vi "Parset_1.vi"(8 "error in (no error)":errorcluster, 11 "Programing Logic in":refnum<class "Programing Logic.lvclass">) -> (0 "error out":errorcluster, 3 "Programing Logic out":refnum<class "Programing Logic.lvclass">)   [LabVIEW 2014, in "Programing Logic.lvclass"]
uses:
  Programing Logic.lvclass
  Programing Logic.lvclass/Programing Logic.ctl
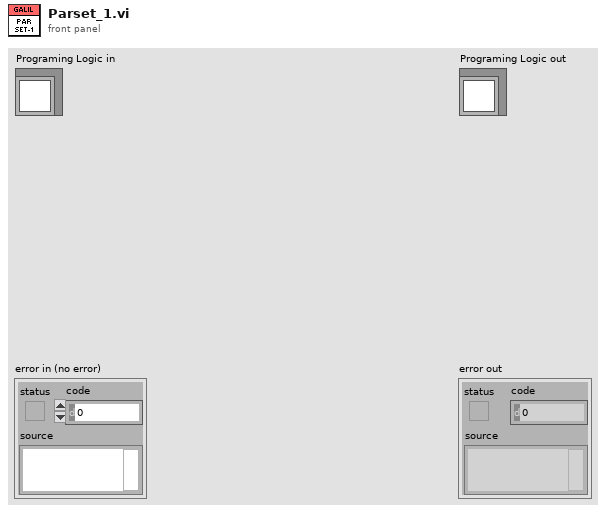
[diagram p1: front panel]
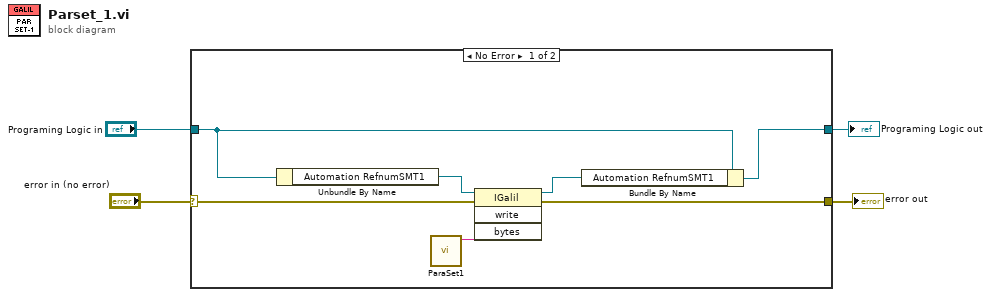
[diagram p0: block diagram]
diagram:
  n1 = case shown="No Error" "error in (no error)" {
    selector: "error in (no error)" -> [w7 w13]
    tunnel: [w6 w13] -> w3
    tunnel: [w9 w12] -> w1
    tunnel: "Programing Logic in" -> [w10 w12]
    frame No Error {
      n2 = Unbundle By Name(w10) -> ("Automation RefnumSMT1"=w11:refnum<k7>)
      n3 = call "ParaSet1.vi"() -> ("String"=w5:string)  [unwired: 11 in]
      n4 = invoke class="IGalil" method="write"(reference=w11, error in=w7, "bytes"=w5) -> (reference out=w8:refnum<k7>, error out=w6:errorcluster)  [unwired: 1 in, 2 out]
      n5 = Bundle By Name(cluster=w10, "Automation RefnumSMT1"=w8) -> (w9:refnum<class "Programing Logic.lvclass">)
    }
    frame Error {
    }
  }
  "error out" <- w3
  "Programing Logic out" <- w1
